vi "FGV_PSP - IPS120 Actions.vi"(4 "error in":errorcluster, 6 "Function":enum16{"write", "read"}(ring), 7 "actions":T1) -> (0 "error out":errorcluster, 3 "actions":T1)   [LabVIEW 2016, in "IPS-120.lvlib" / "IPS-120-API.lvlib"]
uses:
  IPS-120-API.lvlib
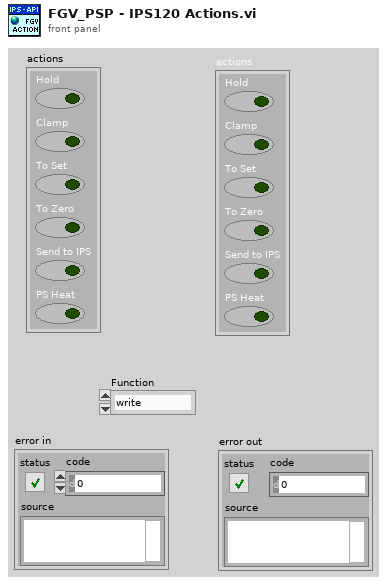
[diagram p1: front panel]
types:
  T1 = cluster{"Hold":bool, "Clamp":bool, "To Set":bool, "To Zero":bool, "Send to IPS":bool, "PS Heat":bool}
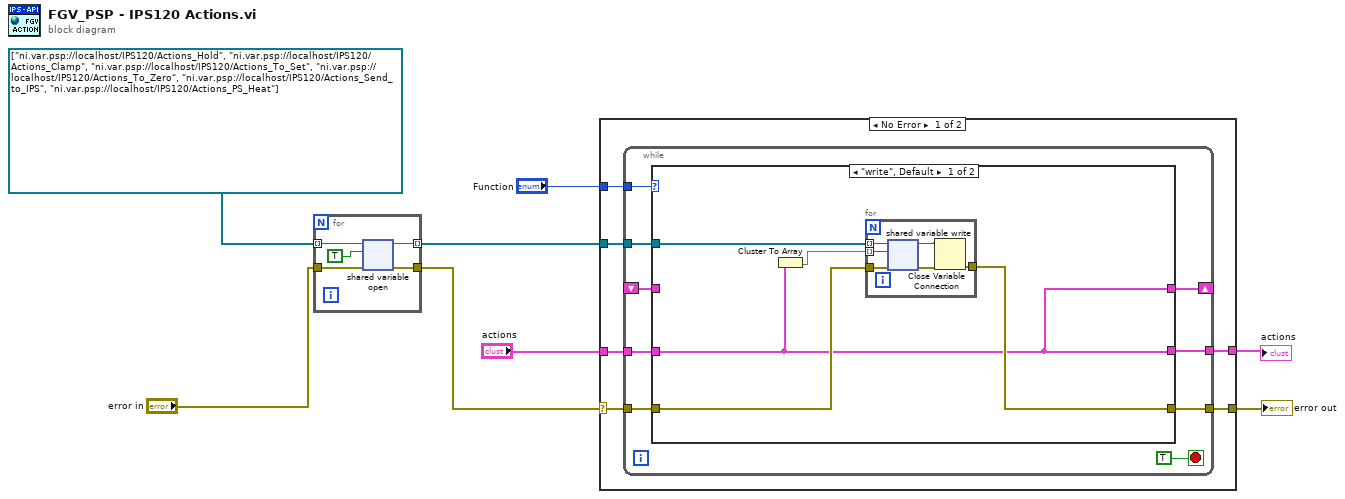
[diagram p0: block diagram]
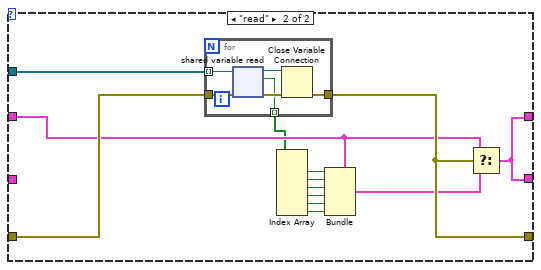
[diagram p2: hidden frame]
diagram:
  n1 = for {
    tunnel: [w13] -> w6 mode=indexing
    tunnel: [w12] -> w5
    tunnel: "error in" -> [w11]
    tunnel: refnum<k21>[] ["ni.var.psp://localhost/IPS120/Actions_Hold", "ni.var.psp://localhost/IPS120/Actions_Clamp", "ni.var.psp://localhost/IPS120/Actions_To_Set", "ni.var.psp://localhost/IPS120/Actions_To_Zero", "ni.var.psp://localhost/IPS120/Actions_Send_to_IPS", "ni.var.psp://localhost/IPS120/Actions_PS_Heat"] -> [w9] mode=indexing
    n2 = shared-variable-open(w9, w11, TRUE) -> (w13:refnum<k21>, w12:errorcluster)  [unwired: 1 in]
  }
  n3 = case shown="No Error" w5 {
    selector: w5 -> [w19 w60]
    tunnel: [w18 w60] -> w8
    tunnel: [w17 w59] -> w1
    tunnel: "Function" -> [w16 _]
    tunnel: w6 -> [w15 _]
    tunnel: "actions" -> [w14 w59]
    frame No Error {
      n4 = while {
        shift-right: [w23] -> _
        shift-left: _ -> [w22]
        tunnel: w19 -> [w27]
        tunnel: [w26] -> w18
        tunnel: [w25] -> w17
        tunnel: w16 -> [w24]
        tunnel: w15 -> [w21]
        tunnel: w14 -> [w20]
        stop <- TRUE stop-if-true
        n5 = case shown="\"write\", Default" w24 {
          tunnel: w27 -> [w32 w50]
          tunnel: [w33 w49] -> w26
          tunnel: [w29 w52] -> w25
          tunnel: [w29 w52] -> w23
          tunnel: w22 -> [_ w48]
          tunnel: w21 -> [w31 w51]
          tunnel: w20 -> [w29 _]
          frame "write", Default {
            n6 = Cluster To Array(cluster=w29) -> (array=w30:bool[])
            n7 = for {
              tunnel: [w38] -> w33
              tunnel: w32 -> [w36]
              tunnel: w31 -> [w35] mode=indexing
              tunnel: w30 -> [w34] mode=indexing
              n8 = shared-variable-write(w35, w36, w34) -> (w37:refnum<k21>, w39:errorcluster)
              n9 = Close Variable Connection(8:w39, 11:w37) -> (0:w38:errorcluster)
            }
          }
          frame "read" {
            n10 = for {
              tunnel: [w56] -> w49
              tunnel: w51 -> [w55] mode=indexing
              tunnel: w50 -> [w54]
              tunnel: [w53] -> w46 mode=indexing
              n11 = shared-variable-read(w55, w54) -> (w58:refnum<k21>, w57:errorcluster, w53:bool)  [unwired: 1 out]
              n12 = Close Variable Connection(8:w57, 11:w58) -> (0:w56:errorcluster)
            }
            n13 = Index Array(array=w46) -> (element #1=w45:bool, element #2=w44:bool, element #3=w43:bool, element #4=w42:bool, element #5=w41:bool, element #6=w40:bool)  [unwired: 6 in]
            n14 = Bundle(cluster=w48, "Hold"=w45, "Clamp"=w44, "To Set"=w43, "To Zero"=w42, "Send to IPS"=w41, "PS Heat"=w40) -> (w47:T1)
            n15 = Select(t=w48, s=w49, f=w47) -> (s? t:f=w52:T1)
          }
        }
      }
    }
    frame Error {
    }
  }
  "error out" <- w8
  "actions" <- w1
